vi "ge_StrainEnum2Ring.vi"(5 "Bridge Type":u16) -> (2 "Bridge Config Ring":u16)   [LabVIEW 2018]
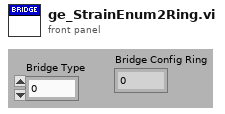
[diagram p1: front panel]
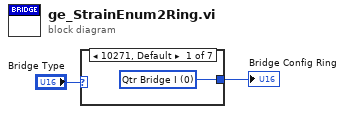
[diagram p0: block diagram]
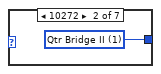
[diagram p2: hidden frame]
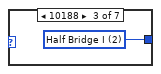
[diagram p3: hidden frame]
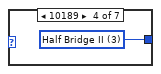
[diagram p4: hidden frame]
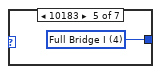
[diagram p5: hidden frame]
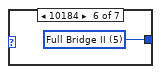
[diagram p6: hidden frame]
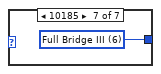
[diagram p7: hidden frame]
diagram:
  n1 = case shown="10271, Default" "Bridge Type" {
    tunnel: [w3 w4 w5 w6 w7 w8 w9] -> w2
    frame 10271, Default {
      w3 = u16 0 items=["Qtr Bridge I", "Qtr Bridge II", "Half Bridge I", "Half Bridge II", "Full Bridge I", "Full Bridge II", "Full Bridge III"] ("Bridge Configuration\n(3:Half Bridge II)")
    }
    frame 10272 {
      w4 = u16 1 items=["Qtr Bridge I", "Qtr Bridge II", "Half Bridge I", "Half Bridge II", "Full Bridge I", "Full Bridge II", "Full Bridge III"] ("Bridge Configuration\n(3:Half Bridge II)")
    }
    frame 10188 {
      w5 = u16 2 items=["Qtr Bridge I", "Qtr Bridge II", "Half Bridge I", "Half Bridge II", "Full Bridge I", "Full Bridge II", "Full Bridge III"] ("Bridge Configuration\n(3:Half Bridge II)")
    }
    frame 10189 {
      w6 = u16 3 items=["Qtr Bridge I", "Qtr Bridge II", "Half Bridge I", "Half Bridge II", "Full Bridge I", "Full Bridge II", "Full Bridge III"] ("Bridge Configuration\n(3:Half Bridge II)")
    }
    frame 10183 {
      w7 = u16 4 items=["Qtr Bridge I", "Qtr Bridge II", "Half Bridge I", "Half Bridge II", "Full Bridge I", "Full Bridge II", "Full Bridge III"] ("Bridge Configuration\n(3:Half Bridge II)")
    }
    frame 10184 {
      w8 = u16 5 items=["Qtr Bridge I", "Qtr Bridge II", "Half Bridge I", "Half Bridge II", "Full Bridge I", "Full Bridge II", "Full Bridge III"] ("Bridge Configuration\n(3:Half Bridge II)")
    }
    frame 10185 {
      w9 = u16 6 items=["Qtr Bridge I", "Qtr Bridge II", "Half Bridge I", "Half Bridge II", "Full Bridge I", "Full Bridge II", "Full Bridge III"] ("Bridge Configuration\n(3:Half Bridge II)")
    }
  }
  "Bridge Config Ring" <- w2
